vi "State_Machine.vi"(8 "error in (no error)":errorcluster caption="entrée d'erreur (pas d'erreur)", 11 "Get_Voltage en entrée":refnum<class "Zigbee_Send_Msg.lvclass">) -> (0 "error out":errorcluster caption="sortie d'erreur", 2 "Json_String":string, 3 "Get_Voltage en sortie":refnum<class "Zigbee_Send_Msg.lvclass">)   [LabVIEW 2020, in "Library Test.lvlib" / "Zigbee_Send_Msg.lvclass"]
uses:
  Zigbee_Send_Msg.lvclass
  C:/Users/ngarcin/OneDrive - Altyor/Standard TB/Suite TB45/Class/Test/Test (Default)/Test (Default).lvclass
  C:/Users/ngarcin/OneDrive - Altyor/Standard TB/Suite TB45/Class/Test/Zigbee_Send_Command_UART/Zigbee_Send_Command_UART.lvclass
  Commun VI/TypeDef/Variable Printable.ctl
  Zigbee_Send_Command_UART/Zigbee_Send_Command_UART.lvclass
  Commun VI/Library Commun.lvlib
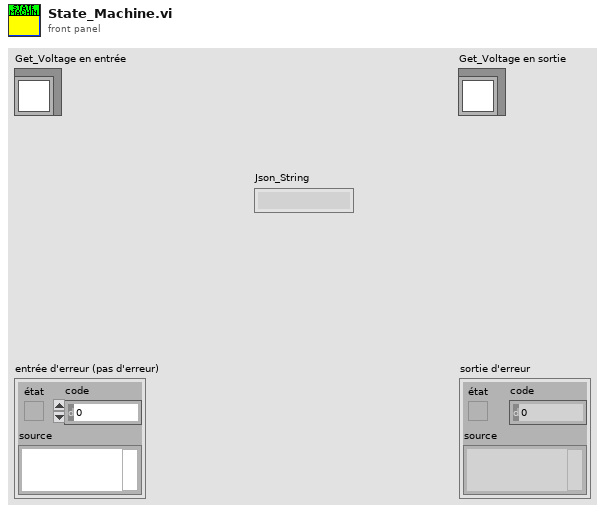
[diagram p1: front panel]
types:
  T1 = typedef "Variable Printable.ctl" = string
  T2 = enum16{"Get Variable", "Get All Variables", "Set Variable", "Delete Variable", "Delete All Variable"}
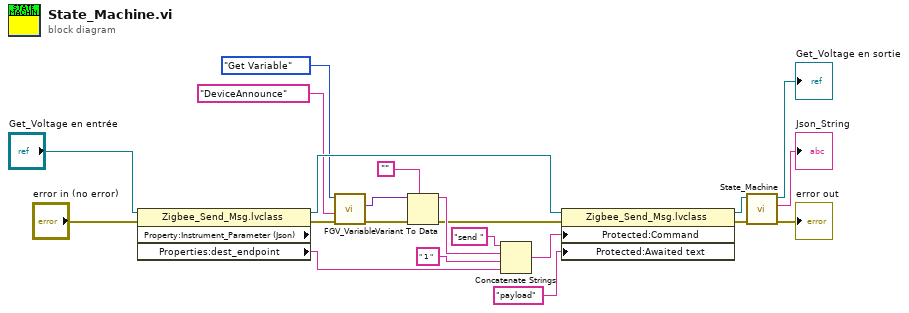
[diagram p0: block diagram]
diagram:
  n1 = property class="Zigbee_Send_Msg.lvclass" props=["Property:Instrument_Parameter (Json)", "Properties:dest_endpoint"](reference="Get_Voltage en entrée", error in="error in (no error)") -> (reference out=w14:refnum<class "Zigbee_Send_Msg.lvclass">, error out=w9:errorcluster, "Properties:dest_endpoint"=w2:string)  [unwired: 1 out]
  n2 = call "FGV_Variable.vi"("error in (no error)"=w9, "Variable"=T1 "DeviceAnnounce", "Function"=T2."Get Variable") -> ("error out"=w8:errorcluster, "Data Out"=w7:variant)  [unwired: 6 in, 1 out]
  n3 = Variant To Data(error in=w8, type="", Variant=w7) -> (data=w5:string, error out=w4:errorcluster)
  n4 = Concatenate Strings("send " ("Command"), w5, " 1 " ("chaîne"), w2) -> (w12:string)
  n5 = property class="Zigbee_Send_Msg.lvclass"(reference=w14, error in=w4, "Protected:Command"=w12, "Protected:Awaited text"="payload" ("Awaited text")) -> (reference out=w18:refnum<class "Zigbee_Send_Msg.lvclass">, error out=w17:errorcluster)
  n6 = call-parent "State_Machine.vi"("error in (no error)"=w17, "Send_Frame en entrée"=w18) -> ("error out"=→"error out":errorcluster, "Json_String"=→"Json_String":string, "Send_Frame en sortie"=→"Get_Voltage en sortie":refnum<class "Zigbee_Send_Msg.lvclass">)  [unwired: 7 in]
